vi "Pareto Inverse CDF.vi"(9 "c":dbl=3.0, 10 "a":dbl=1.0, 11 "cdf(x)":dbl=0.1) -> (0 "error":i32, 3 "x":dbl=1.0357441686512863)   [LabVIEW 2017, in "NI_Gmath.lvlib"]
doc: "Computes the continuous inverse cumulative distribution function (CDF) of the various distributions. You must manually select the polymorphic instance to use."
uses:
  NI_Gmath.lvlib
  st_error_code.ctl
panel:
  # "Pareto Inverse CDF"
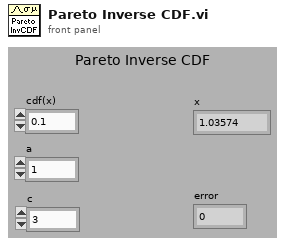
[diagram p1: front panel]
types:
  T1 = typedef "NI_Gmath.lvlib/st_error_code.ctl" = i32
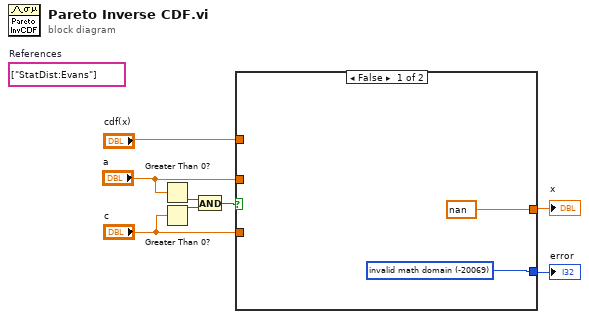
[diagram p0: block diagram]
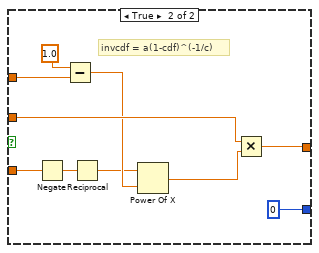
[diagram p2: hidden frame]
diagram:
  (unwired) string[] ["StatDist:Evans"]  # References
  n1 = Greater Than 0?(x="a") -> (x > 0?=w3:bool)
  n2 = Greater Than 0?(x="c") -> (x > 0?=w2:bool)
  n3 = And(x=w3, y=w2) -> (x .and. y?=w1:bool)
  n4 = case shown="False" w1 {
    tunnel: "c" -> [_ w13]
    tunnel: [w9 0 ("invalid math domain")] -> w7
    tunnel: [nan w11] -> w8
    tunnel: "cdf(x)" -> [_ w18]
    tunnel: "a" -> [_ w17]
    frame False {
      w9 = T1 -20069 items=["invalid math domain"=-20069, "Fourier interpolation size m >= n"=-20070, "empty array"=-20003] ("stat interp error code")
    }
    frame True {
      # "invcdf = a(1-cdf)^(-1/c)"
      n5 = Negate(x=w13) -> (-x=w14:dbl)
      n6 = Subtract(x=1.0, y=w18) -> (x-y=w15:dbl)
      n7 = Reciprocal(x=w14) -> (1/x=w12:dbl)
      n8 = Power Of X(1:w15, 2:w12) -> (0:w16:dbl)
      n9 = Multiply(x=w17, y=w16) -> (x*y=w11:dbl)
    }
  }
  "x" <- w8
  "error" <- w7
